vi "生成CODMn data (子VI).vi"() -> (3 "data":T1)   [LabVIEW 2016, in "斯坦道CODMn.lvlib"]
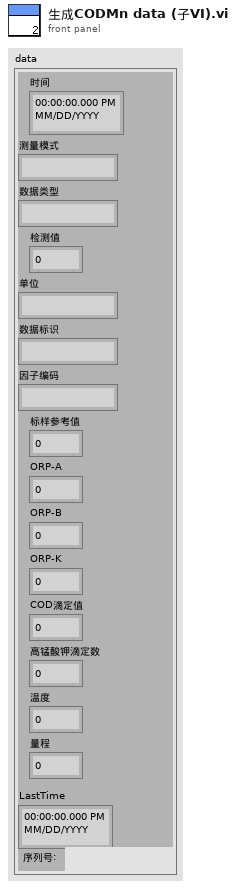
[diagram p1: front panel]
types:
  T1 = cluster{"时间":timestamp, "测量模式":string, "数据类型":string, "检测值":sgl, "单位":string, "数据标识":string, "因子编码":string, "标样参考值":sgl, "ORP-A":sgl, "ORP-B":sgl, "ORP-K":sgl, "COD滴定值":sgl, "高锰酸钾滴定数":sgl, "温度":sgl, "量程":sgl, "LastTime":timestamp, "序列号:":string}
  T2 = cluster{"运行模式":enum16{"维护模式", "常规模式", "应急模式", "质控模式"}, "质控频次":enum16{"关闭", "每天", "星期一", "星期二", "星期三", "星期四", "星期五", "星期六", "星期日"}, "空白核查时间":u16, "跨度核查时间":u16, "24H周期设置":bool[]}
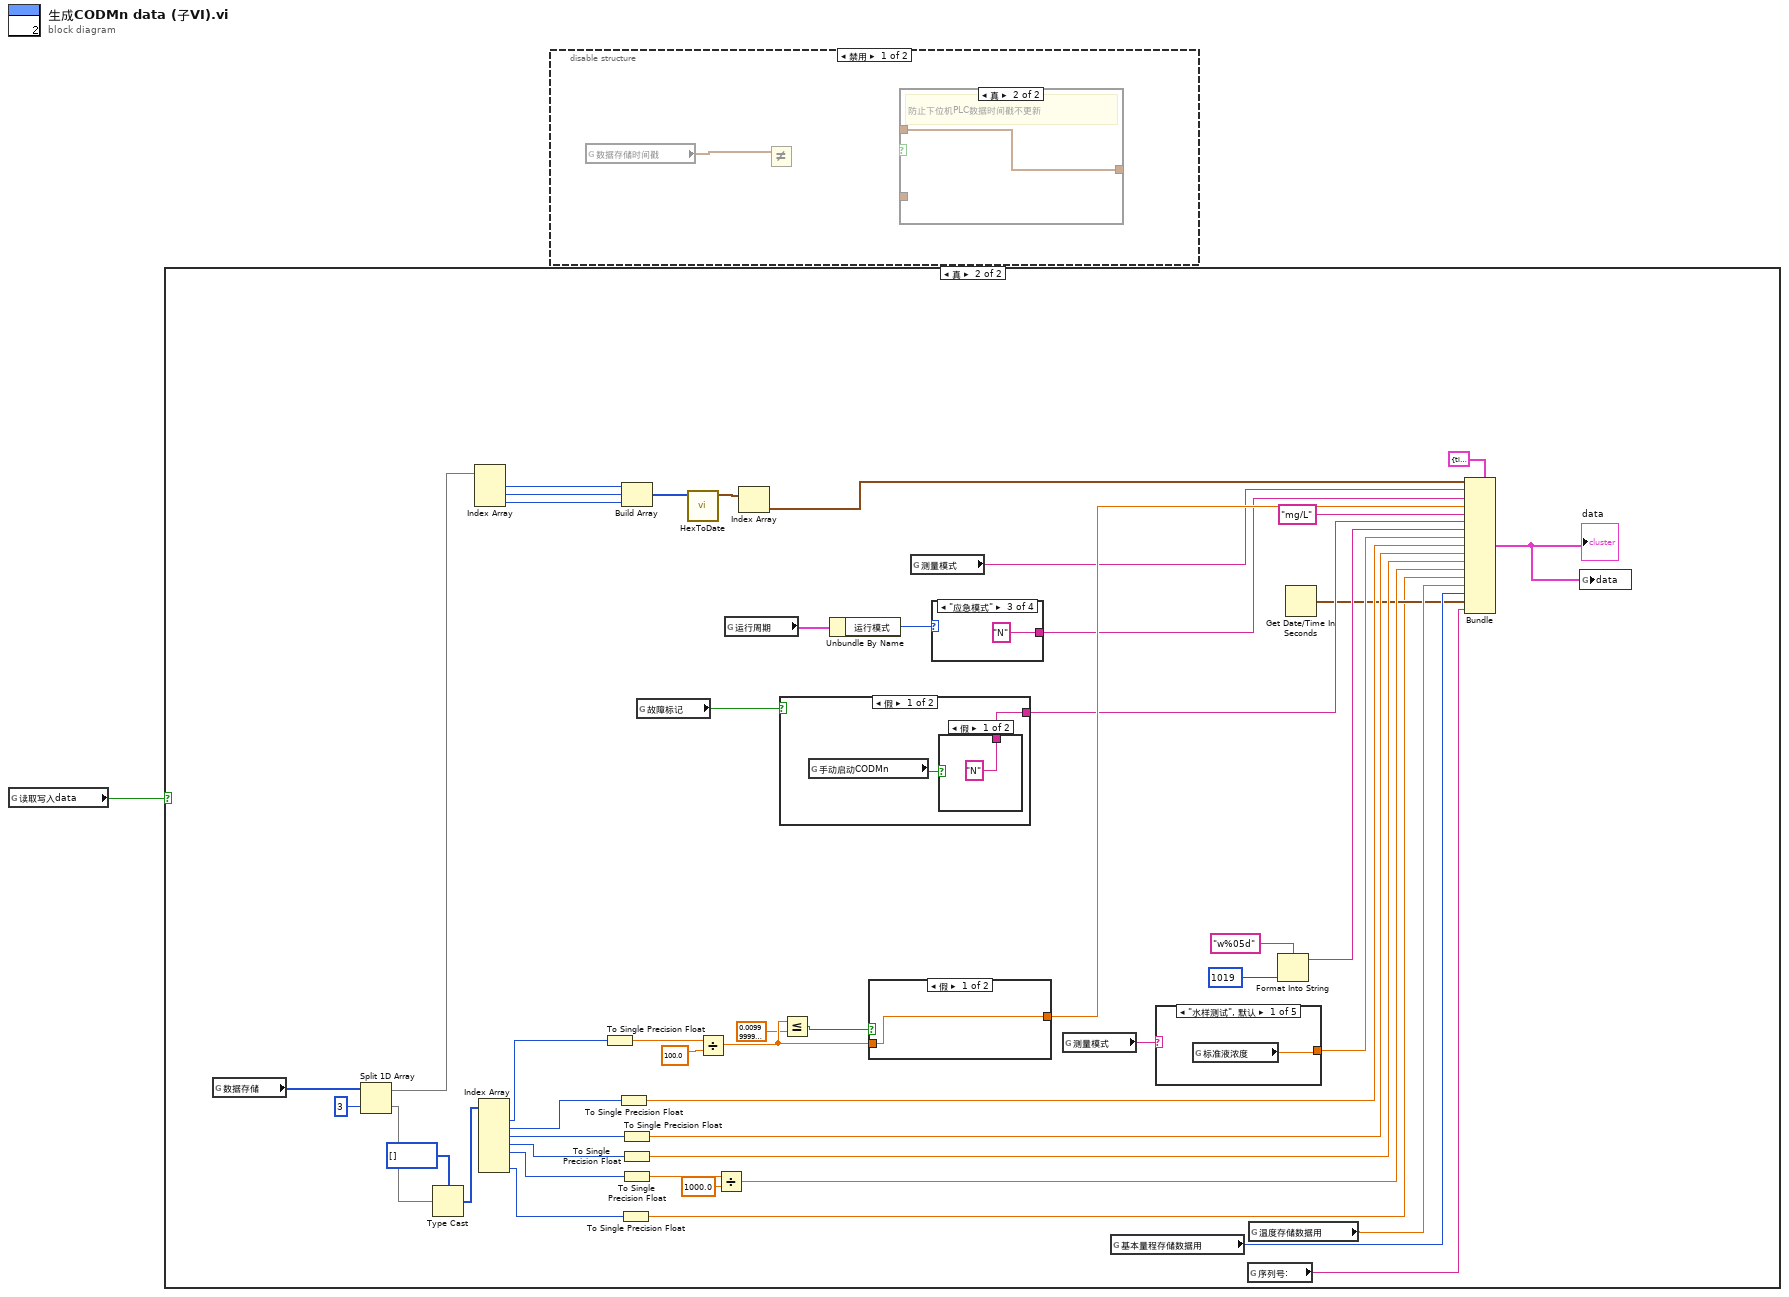
[diagram p0: block diagram]
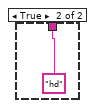
[diagram p5: hidden frame]
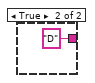
[diagram p6: hidden frame]
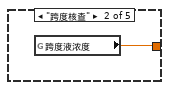
[diagram p7: hidden frame]
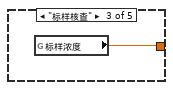
[diagram p8: hidden frame]
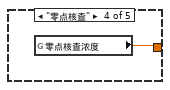
[diagram p9: hidden frame]
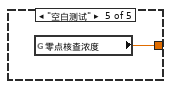
[diagram p10: hidden frame]
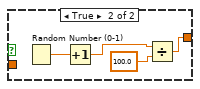
[diagram p11: hidden frame]
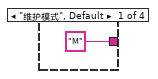
[diagram p12: hidden frame]
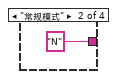
[diagram p13: hidden frame]
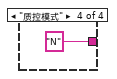
[diagram p14: hidden frame]
diagram:
  n1 = global read "COD内部交互全局.vi" "读取写入data"() -> (w1:bool)
  n2 = case shown="真" w1 {
    frame False {
    }
    frame True {
      n3 = global read "COD内部交互全局.vi" "数据存储"() -> (w11:u16[])
      n4 = Split 1D Array(array=w11, index=3 ("索引")) -> (first subarray=w16:u16[], second subarray=w10:u16[])
      n5 = Type Cast(type=i16[] [], x=w10) -> (*(type *) &x=w9:i16[])
      n6 = Index Array(array=w16) -> (element #1=w18:u16, element #2=w19:u16, element #3=w20:u16)  [unwired: 3 in]
      n7 = Index Array(array=w9) -> (element #1=w43:i16, element #2=w22:i16, element #3=w23:i16, element #4=w24:i16, element #5=w25:i16, element #7=w48:i16)  [unwired: 7 in, 1 out]
      n8 = To Single Precision Float(number=w43) -> (single precision float=w41:sgl)
      n9 = To Single Precision Float(number=w22) -> (single precision float=w34:sgl)
      n10 = To Single Precision Float(number=w48) -> (single precision float=w8:sgl)
      n11 = Build Array(w18, w19, w20) -> (w21:u16[])
      n12 = To Single Precision Float(number=w23) -> (single precision float=w33:sgl)
      n13 = To Single Precision Float(number=w24) -> (single precision float=w32:sgl)
      n14 = To Single Precision Float(number=w25) -> (single precision float=w28:sgl)
      n15 = global read "COD内部交互全局.vi" "故障标记"() -> (w50:bool)
      n16 = call "HexToDate.vi"("数组"=w21) -> ("DATE"=w17:timestamp[])  [unwired: 10 in]
      n17 = Divide(x=w41, y=sgl 100.0) -> (x/y=w42:sgl)
      n18 = Divide(x=w28, y=sgl 1000.0) -> (x/y=w31:sgl)
      n19 = global read "CODMn断电保存全局变量.vi" "运行周期"() -> (w3:T2)
      n20 = Index Array(array=w17) -> (element=w7:timestamp)  [unwired: 1 in]
      n21 = case shown="假" w50 {
        tunnel: [w52 "D" ("数据标识")] -> w36
        frame False {
          n22 = global read "CODMN外部API.vi" "手动启动CODMn"() -> (w51:bool)
          n23 = case shown="假" w51 {
            tunnel: ["N" ("数据标识") "hd" ("数据标识")] -> w52
            frame False {
            }
            frame True {
            }
          }
        }
        frame True {
        }
      }
      n24 = Less Or Equal?(x=w42, y=sgl 0.01) -> (x <= y?=w40:bool)
      n25 = Unbundle By Name(w3) -> ("运行模式"=w2:enum16{"维护模式", "常规模式", "应急模式", "质控模式"})
      n26 = case shown="假" w40 {
        tunnel: [w61 w62] -> w47
        tunnel: w42 -> [w61 _]
        frame False {
        }
        frame True {
          n27 = Random Number (0-1)() -> (number: 0 to 1=w65:dbl)
          n28 = Increment(x=w65) -> (x+1=w63:dbl)
          n29 = Divide(x=w63, y=sgl 100.0) -> (x/y=w62:dbl)
        }
      }
      n30 = global read "COD测量模式全局.vi" "测量模式"() -> (w46:string)
      n31 = case shown="\"应急模式\"" w2 {
        tunnel: ["M" ("单位") "N" ("单位") "N" ("单位") "N" ("单位")] -> w38
        frame "维护模式", Default {
        }
        frame "常规模式" {
        }
        frame "应急模式" {
        }
        frame "质控模式" {
        }
      }
      n32 = global read "COD测量模式全局.vi" "测量模式"() -> (w44:string)
      n33 = global read "COD内部交互全局.vi" "基本量程存储数据用"() -> (w14:enum16{"L", "H", "AUTO"})
      n34 = case shown="\"水样测试\", 默认" w44 {
        tunnel: [w56 w57 w58 w59 w60] -> w45
        frame "水样测试", Default {
          n35 = global read "COD浓度全局变量.vi" "标准液浓度"() -> (w56:dbl)
        }
        frame "跨度核查" {
          n36 = global read "CODMn断电保存全局变量.vi" "跨度液浓度"() -> (w57:dbl)
        }
        frame "标样核查" {
          n37 = global read "CODMn断电保存全局变量.vi" "标样浓度"() -> (w58:dbl)
        }
        frame "零点核查" {
          n38 = global read "CODMn断电保存全局变量.vi" "零点核查浓度"() -> (w59:dbl)
        }
        frame "空白测试" {
          n39 = global read "CODMn断电保存全局变量.vi" "零点核查浓度"() -> (w60:dbl)
        }
      }
      n40 = global read "COD内部交互全局.vi" "序列号:"() -> (w5:string)
      n41 = global read "COD内部交互全局.vi" "温度存储数据用"() -> (w49:dbl)
      n42 = Format Into String(format string="w%05d" ("格式字符串"), u32 1019 ("因子编码")) -> (resulting string=w35:string)  [unwired: 2 in, 1 out]
      n43 = Get Date/Time In Seconds() -> (seconds since 1Jan1904=w13:timestamp)
      n44 = Bundle(cluster=T1 {"时间"=timestamp(0 s since 1904-01-01), "测量模式"="", "数据类型"="", "检测值"=0.0, "单位"="", "数据标识"="", "因子编码"="", "标样参考值"=0.0, "ORP-A"=0.0, "ORP-B"=0.0, "ORP-K"=0.0, "COD滴定值"=0.0, "高锰酸钾滴定数"=0.0, "温度"=0.0, "量程"=0.0, "LastTime"=timestamp(0 s since 1904-01-01), "序列号:"=""} ("data"), "时间"=w7, "测量模式"=w46, "数据类型"=w38, "检测值"=w47, "单位"="mg/L", "数据标识"=w36, "因子编码"=w35, "标样参考值"=w45, "ORP-A"=w34, "ORP-B"=w33, "ORP-K"=w32, "COD滴定值"=w31, "高锰酸钾滴定数"=w8, "温度"=w49, "量程"=w14, "LastTime"=w13, "序列号:"=w5) -> (w4:T1)
      "data" <- w4
      n45 = global write "COD内部交互全局.vi" "data"(w4) -> ()
    }
  }
  n46 = disable-structure shown="禁用" {
    frame Disabled {
      n47 = global read "COD内部交互全局.vi" "数据存储时间戳"() -> (w70:timestamp)
      n48 = Not Equal?(x=w70) -> (x != y?=w71:bool)  [unwired: 1 in]
      n49 = case "条件结构" shown="真" {
        selector: _ -> [_ _]
        tunnel: _ -> [w72 _]
        tunnel: _ -> [_ w73]
        tunnel: [w72 w73] -> _
        frame False {
        }
        frame True {
          # "防止下位机PLC数据时间戳不更新"
        }
      }
    }
    frame Enabled {
    }
  }
